vi "LoadNodeUI.vi"(7 "user event out":T1, 8 "error in":errorcluster, 9 "sub panel ref in":refnum<vi>, 10 "main queue":T3, 11 "node":T2) -> (0 "error out":errorcluster)   [LabVIEW 2013, in "NISE_CEF_TreeControl.lvlib"]
doc: "This VI will insert the UI from a node into a subpanel."
uses:
  NISE_CEF_TreeControl.lvlib
  <vilib>/NI/AMC/Message Queue.ctl
  <vilib>/NI/AMC/Message.ctl
  <vilib>/NI/Tools/Keyed Array/KeyedArray.ctl
  Node/NodeRef.ctl
  Node/NISE_CEF_Node.lvclass
  Node/UserEventRef.ctl
  Controls/EventCluster.ctl
  <vilib>/NI/Tools/Keyed Array/Tools_KeyedArray.lvlib
  <vilib>/NI/AMC/AMC.lvlib
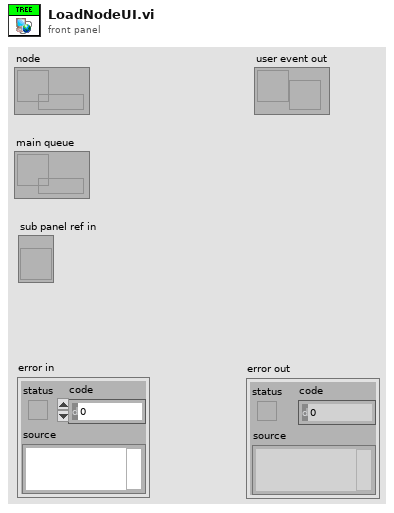
[diagram p1: front panel]
types:
  T1 = typedef "NISE_CEF_Node.lvclass/UserEventRef.ctl" = refnum<user-event>
  T2 = typedef "NISE_CEF_Node.lvclass/NodeRef.ctl" = refnum<data-value>
  T3 = typedef "AMC.lvlib/Message Queue.ctl" = refnum<queue>
  T4 = enum32{"Bad", "Idle", "Run top level", "Running"}
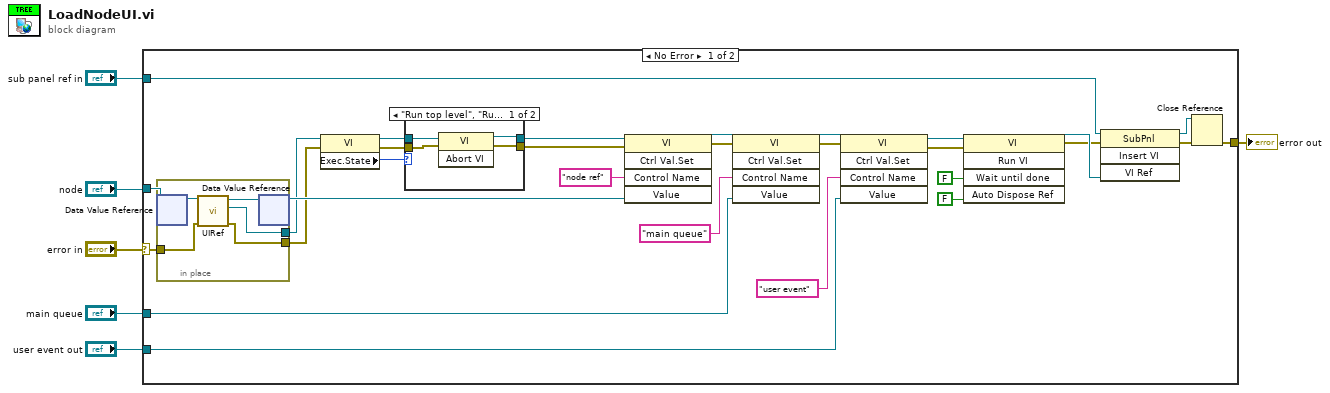
[diagram p0: block diagram]
diagram:
  n1 = case shown="No Error" "error in" {
    selector: "error in" -> [w18 w47]
    tunnel: [w25 w47] -> w5
    tunnel: "node" -> [w10 _]
    tunnel: "main queue" -> [w9 _]
    tunnel: "user event out" -> [w8 _]
    tunnel: "sub panel ref in" -> [w7 _]
    frame No Error {
      n2 = in-place {
        in-place-border: w18 -> [w43]
        in-place-border: [w44] -> w17
        in-place-border: [w42] -> w13
        n3 = in-place-dvr #1(w10) -> (w46:refnum<class "NISE_CEF_Node.lvclass">)  [unwired: 1 out]
        n4 = call-dynamic "UIRef.vi"("error in"=w43, "node in"=w46) -> ("error out"=w42:errorcluster, "VI refnum"=w44:refnum<vi>, "node out"=w45:refnum<class "NISE_CEF_Node.lvclass">)  [unwired: 7 in]
        n5 = in-place-dvr #1(w45) -> (w19:T2)  [unwired: 1 out]
      }
      n6 = property class="VI"(reference=w17, error in=w13) -> (reference out=w14:refnum<vi>, error out=w12:errorcluster, "Exec.State"=w16:T4)
      n7 = case shown="\"Run top level\", \"Running\"" w16 {
        tunnel: [w36 w41] -> w15
        tunnel: w14 -> [w39 w41]
        tunnel: w12 -> [w38 w40]
        tunnel: [w37 w40] -> w11
        frame "Run top level", "Running" {
          n8 = invoke class="VI" method="Abort VI"(reference=w39, error in=w38) -> (reference out=w36:refnum<vi>, error out=w37:errorcluster)  [unwired: 1 in, 1 out]
        }
        frame "Idle", Default {
        }
      }
      n9 = invoke class="VI" method="Ctrl Val.Set"(reference=w15, error in=w11, "Control Name"="node ref", "Value"=w19) -> (reference out=w33:refnum<vi>, error out=w28:errorcluster)  [unwired: 1 in, 3 out]
      n10 = invoke class="VI" method="Ctrl Val.Set"(reference=w33, error in=w28, "Control Name"="main queue", "Value"=w9) -> (reference out=w23:refnum<vi>, error out=w24:errorcluster)  [unwired: 1 in, 3 out]
      n11 = invoke class="VI" method="Ctrl Val.Set"(reference=w23, error in=w24, "Control Name"="user event", "Value"=w8) -> (reference out=w22:refnum<vi>, error out=w21:errorcluster)  [unwired: 1 in, 3 out]
      n12 = invoke class="VI" method="Run VI"(reference=w22, error in=w21, "Wait until done"=FALSE ("Wait Until Done"), "Auto Dispose Ref"=FALSE ("Auto Dispose Reference")) -> (reference out=w32:refnum<vi>, error out=w31:errorcluster)  [unwired: 1 in, 3 out]
      n13 = invoke class="SubPnl" method="Insert VI"(reference=w7, error in=w31, "VI Ref"=w32) -> (reference out=w26:refnum<vi>, error out=w27:errorcluster)  [unwired: 1 in, 2 out]
      n14 = Close Reference(reference=w26, error in (no error)=w27) -> (error out=w25:errorcluster)
    }
    frame Error {
    }
  }
  "error out" <- w5
